vi "Get Module Type.vi"(8 "error in (no error)":errorcluster, 11 "Module in":refnum<class "Module.lvclass">) -> (0 "error out":errorcluster, 2 "Type":string, 3 "Module out":refnum<class "Module.lvclass">)   [LabVIEW 2019, in "Module.lvclass"]
uses:
  Module.lvclass
  Module Configuration.ctl
  Module.lvclass/Module.ctl
  VI/Module Loop/Module Loop.lvclass
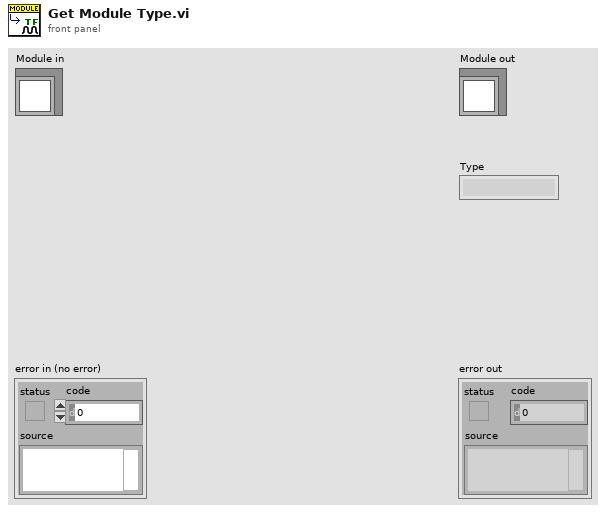
[diagram p1: front panel]
types:
  T1 = typedef "Module Loop.lvclass/Module Configuration.ctl" = cluster{"Type":string, "Direction":string, "Speed":string, "Channels":string, "FXP Type":string}
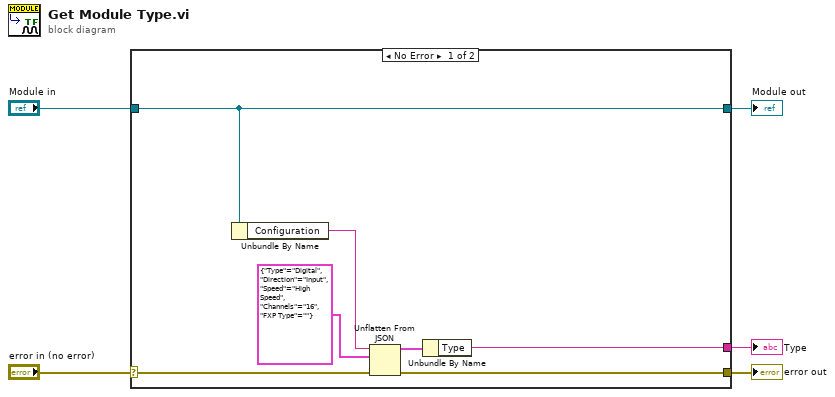
[diagram p0: block diagram]
diagram:
  n1 = case shown="No Error" "error in (no error)" {
    selector: "error in (no error)" -> [w10 w14]
    tunnel: [w9 w14] -> w4
    tunnel: [w12 w13] -> w2
    tunnel: "Module in" -> [w12 w13]
    tunnel: [w6 _] -> w1
    frame No Error {
      n2 = Unbundle By Name(w12) -> ("Configuration"=w11:string)
      n3 = Unflatten From JSON(JSON string=w11, type and defaults=T1 {"Type"="Digital", "Direction"="Input", "Speed"="High Speed", "Channels"="16", "FXP Type"=""} ("Cluster"), error in (no error)=w10) -> (value=w7:T1, error out=w9:errorcluster)  [unwired: 4 in]
      n4 = Unbundle By Name(w7) -> ("Type"=w6:string)
    }
    frame Error {
    }
  }
  "error out" <- w4
  "Module out" <- w2
  "Type" <- w1
